vi "Generation Test.vi"   [LabVIEW 2014]
uses:
  <vilib>/Platform/TimedLoop/XDataNode/timing_clust.ctl
  <vilib>/Platform/TimedLoop/XDataNode/nitl_modes.ctl
  <vilib>/Platform/TimedLoop/XDataNode/wakeup.ctl
  <vilib>/rvi/eio/common/nirviEmuTemplateMethod_errors.vi
  <vilib>/rvi/Emulation/niFpgaSctlEmulationGetInTimedLoop.vi
  <vilib>/rvi/Emulation/niFpgaEmulationReportErrorSimple.vi
  <vilib>/rvi/Emulation/niFpgaGetClockAttributes.vi
  <vilib>/rvi/Emulation/niFpgaCriticalErrorInLSC.vi
  <vilib>/rvi/Memory/Memory_Emulation/nirvimemoryEmulation.vi
  <vilib>/rvi/Memory/Memory_Emulation/nirvimemoryFastEmulation.vi
  <vilib>/rvi/DataTransferAndStorage/Container/Common/niFpgaContainerGetUniqueNameForEmu.vi
  <vilib>/rvi/Memory/Memory_Emulation/niFpgaMemoryEmulationCacheClearOnFirstRun.vi
  <vilib>/rvi/Memory/Memory_Emulation/nirvimemoryEmulationManagerCache_MakeExclusive.vi
  <vilib>/rvi/Memory/Memory_Emulation/niFpgaMemoryEmulationValidateCache.vi
  <vilib>/rvi/Memory/Memory_Emulation/nirvimemoryEmulationManagerCache_InsertValue.vi
  <vilib>/Utility/error.llb/Clear Errors.vi
  <vilib>/rvi/Memory/Memory_Emulation/nirvimemoryEmulationManagerCache_ReleaseExclusive.vi
  <vilib>/rvi/Memory/Memory_Emulation/nirvimemoryEmulationManagerCache_GetValue.vi
  <vilib>/rvi/Emulation/niFpgaEmulationIsFPGAContextNoSignature.vi
  <vilib>/rvi/Memory/Memory_Emulation/nirvimemoryEmulationManagerCache_SetValue.vi
  <vilib>/rvi/Emulation/niFpgaSctlEmulationResourceMgr.vi
  <vilib>/rvi/errors/niFpgaSetErrorForExecOnDevCompSimple.vi
  <vilib>/rvi/eio/common/nirviEmuReportErrorAndStop.vi
  <vilib>/rvi/FIFO/Fifo_Resource/nirvififoEmulationSetSize.vi
  <vilib>/rvi/FIFO/Fifo_Resource/nirviFifoEmulationQueueMgr.vi
  <instcachedir>/0/nirviFifoEmulationQueueMgr_E5CAEC123FF24DC58D834DCA3CDAA9B5.lvgen/nirviFifoEmulationQueueMgr_E5CAEC123FF24DC58D834DCA3CDAA9B5_009.vi
  <vilib>/rvi/FIFO/Fifo_Resource/nirvififoEmulationDetermineInputValidOut.vi
  <vilib>/rvi/FIFO/Fifo_Resource/nirvififoEmulationCreateLock.vi
  <vilib>/rvi/Emulation/niFpgaProcessEmulError.vi
  <vilib>/rvi/FIFO/Fifo_Resource/nirvififoEmulationObtainLock.vi
  <vilib>/rvi/FIFO/Fifo_Resource/nirvififoEmulationReleaseLock.vi
  <vilib>/rvi/occurrence/nirviWaitOnOccurrenceBase.vi
  <vilib>/rvi/errors/nirviReportUnexpectedCaseInternalError.vi
  <vilib>/rvi/errors/nirviReportUnexpectedCaseInternalError (U32).vi
  <vilib>/eio/EIOMethodNode/EIOMethodNode.xnode
  <vilib>/Platform/TimedLoop/XDataNode/XDataNode.xnode
  <vilib>/rvi/DataTransferAndStorage/Container/XNode/niFpgaContainer.xnode
  <vilib>/rvi/FIFO/Fifo_Resource/nirvififoEmulationWrite.vi
  <vilib>/rvi/FIFO/Fifo_Resource/nirvififoEmulationRead.vi
  <vilib>/Platform/TimedLoop/XDataNode/XDNodeRunTimeDep.lvlib
types:
  T1 = typedef "XDNodeRunTimeDep.lvlib/timing_clust.ctl" = cluster{"Expected End [f-1]":u64, "Actual End [f-1]":u64, "Finished Late? [f-1]":bool, "Expected End [i-1]":u64, "Actual End [i-1]":u64, "Finished Late? [i-1]":bool, "Expected Start [i]":u64, "Actual Start [i]":u64, "Expected Start [f]":u64, "Actual Start [f]":u64, "Source Name":string, "Structure Name":string, "Period":i64, "Deadline":i64, "Offset":i64, "Start":i64, "Priority":i32, "Timeout":i32, "Mode":T2, "Wakeup Reason":T3, "Error":errorcluster, "Source Type":string, "Secondary Source Type":string, "Global End Time":u64, "Global Start Time":u64, "Frame Duration":u64, "Iteration Duration":u64, "Assigned CPU":i32, "I/O Scan Engine Mode":u32}
  T2 = typedef "XDNodeRunTimeDep.lvlib/nitl_modes.ctl" = enum32{"No Change", "Process missed periods, maintain original phase", "Discard missed periods, maintain original phase", "Process missed periods, ignore original phase", "Discard missed periods, ignore original phase"}
  T3 = typedef "XDNodeRunTimeDep.lvlib/wakeup.ctl" = enum32{"Normal", "Aborted", "Asynchronous wakeup", "Timing source error", "Timed loop error", "Timeout"}
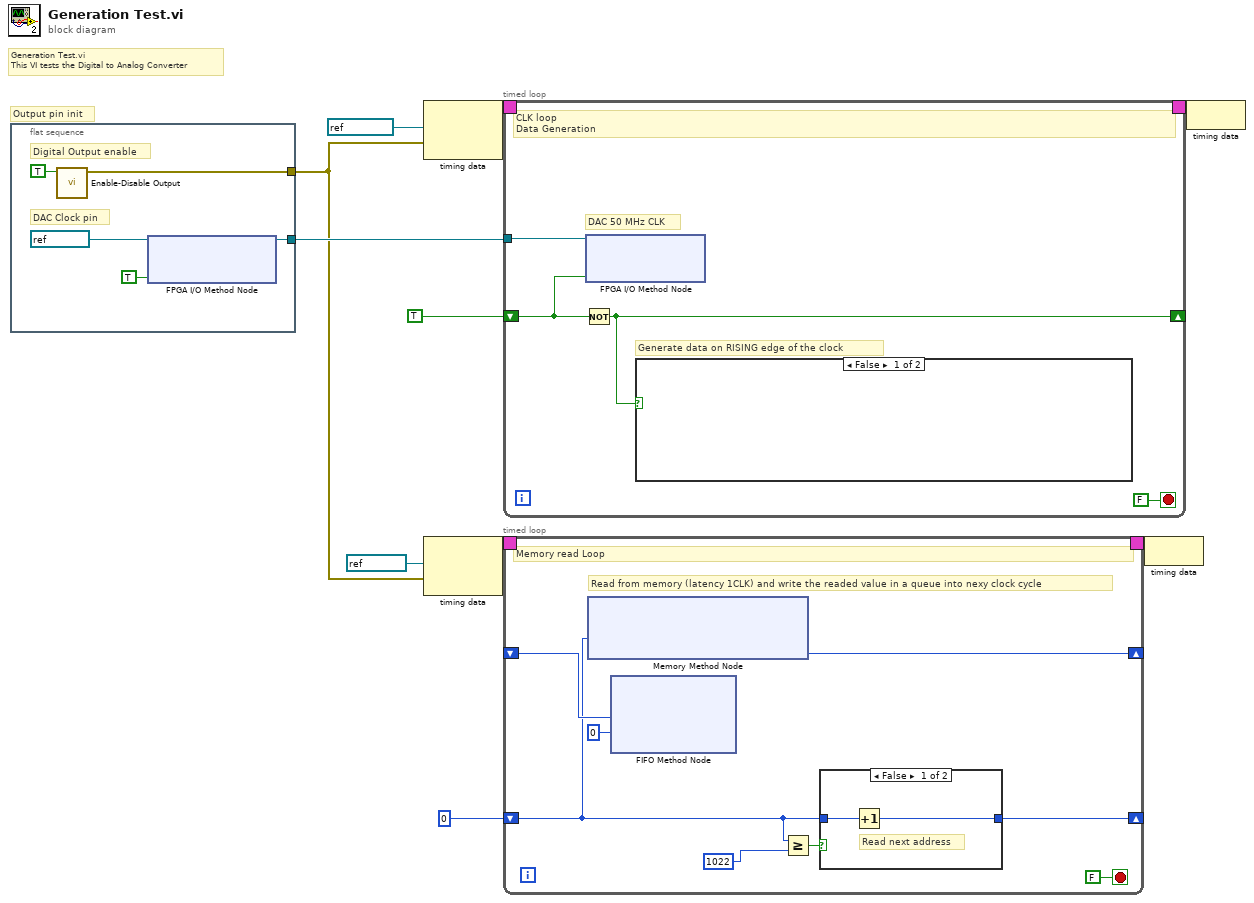
[diagram p0: block diagram]
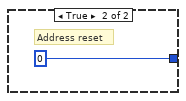
[diagram p2: hidden frame]
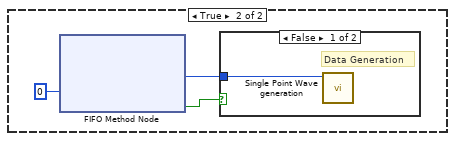
[diagram p3: hidden frame]
diagram:
  # "Generation Test.vi\nThis VI tests the Digital to Analog Converter"
  # "Output pin init"
  n1 = flat-sequence {
    tunnel: [w13] -> w6
    tunnel: [w11] -> w1
    frame #0 {
      # "Digital Output enable"
      # "DAC Clock pin"
      n2 = call "Enable-Disable Output.vi"("Enable"=TRUE) -> ("error out"=w11:errorcluster)  [unwired: 10 in]
      n3 = xnode "FPGA I/O Method Node"("FPGA I/O In"=refnum<k21> "DIO16", "Enable"=TRUE) -> ("FPGA I/O Out"=w13:refnum<k21>)
    }
  }
  n4 = node-c288(refnum<k21> "100MHz" ("Source Name"), w1) -> (w10:T1)
  n5 = node-c288(refnum<k21> "50MHz" ("Source Name"), w1) -> (w5:T1)
  n6 = timed-loop {
    timing: w10 -> [_]
    timing-out: [_] -> w9
    shift-right: [w16] -> _
    shift-left: TRUE -> [w17]
    tunnel: w6 -> [w19]
    stop <- FALSE stop-if-true
    # "Generate data on RISING edge of the clock"
    # "DAC 50 MHz CLK"
    # "CLK loop\nData Generation"
    n7 = Not(x=w17) -> (.not. x?=w16:bool)
    n8 = xnode "FPGA I/O Method Node"("FPGA I/O In"=w19, "Data"=w17) -> ()  [unwired: 1 out]
    n9 = case shown="False" w16 {
      frame False {
      }
      frame True {
        n10 = xnode ("FIFO Method Node")("Timeout"=0) -> ("Element"=w22:i16, "Timed Out?"=w20:bool)  [unwired: 1 in, 1 out]
        n11 = case shown="False" w20 {
          tunnel: w22 -> [w23 _]
          frame False {
            # "Data Generation"
            n12 = call "Single Point Wave generation.vi"("Data To Write"=w23) -> ()  [unwired: 10 in, 1 out]
          }
          frame True {
            # "FPGA memory slow"
          }
        }
      }
    }
  }
  n13 = timed-loop {
    timing: w5 -> [_]
    timing-out: [_] -> w4
    shift-right: [w33] -> _
    shift-left: _ -> [w30]
    shift-right: [w31] -> _
    shift-left: u32 0 -> [w27]
    stop <- FALSE stop-if-true
    # "Read from memory (latency 1CLK) and write the readed value in a queue into nexy clock cycle"
    # "Memory read Loop"
    n14 = xnode ("Memory Method Node")("Address"=w27) -> ("Data"=w33:i16)  [unwired: 1 in, 1 out]
    n15 = xnode ("FIFO Method Node")("Element"=w30, "Timeout"=0) -> ()  [unwired: 1 in, 2 out]
    n16 = Greater Or Equal?(x=w27, y=u32 1022) -> (x >= y?=w32:bool)
    n17 = case shown="False" w32 {
      tunnel: w27 -> [w35 _]
      tunnel: [w34 u32 0] -> w31
      frame False {
        # "Read next address"
        n18 = Increment(x=w35) -> (x+1=w34:u32)
      }
      frame True {
        # "Address reset"
      }
    }
  }
  n19 = node-c288(w4) -> ()
  n20 = node-c288(w9) -> ()
